vi "被测通道数.vi"(1 "被测通道":tag="PXI1Slot3/ai1" caption="标准通道") -> (0 "被测通道数":i32)   [LabVIEW 2015]
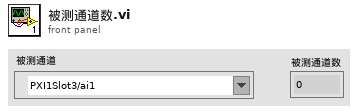
[diagram p1: front panel]
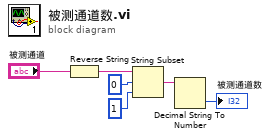
[diagram p0: block diagram]
diagram:
  n1 = Reverse String(1:"被测通道") -> (0:w5:string)
  n2 = String Subset(string=w5, offset (0)=0 ("偏移量(0)"), length (rest)=1 ("长度（剩余）")) -> (substring=w2:string)
  n3 = Decimal String To Number(string=w2) -> (number=→"被测通道数":i32)  [unwired: 2 in, 1 out]
